vi "Create XY Graph (subVI).vi"(8 "error in":errorcluster caption="error in (no error)", 10 "Direction":dbl[](array[numeric]), 11 "Magnitude":dbl[](array[numeric])) -> (0 "error out":errorcluster, 1 "Polar Array":cluster{dbl, dbl}[](array[cluster]), 3 "XY Graph":cluster{"Y":dbl[], "Y":dbl[]}[](graph))   [LabVIEW 2016]
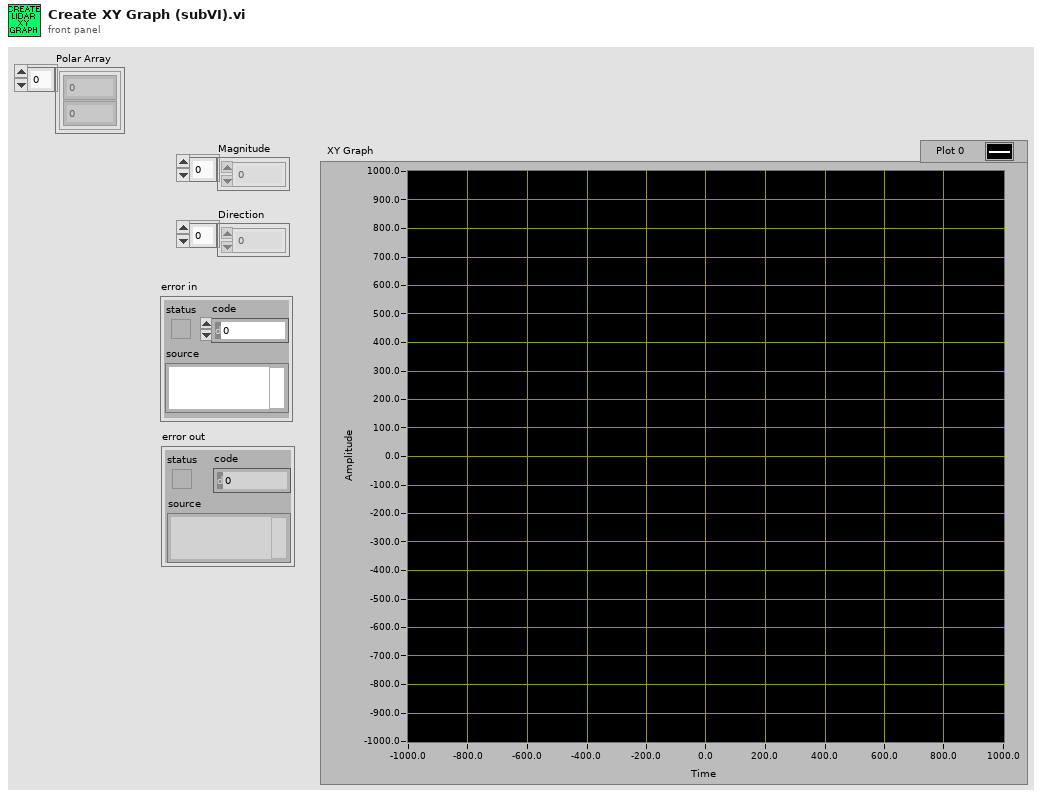
[diagram p1: front panel]
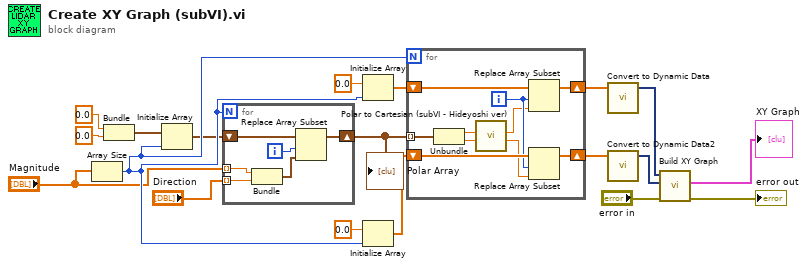
[diagram p0: block diagram]
diagram:
  n1 = Array Size(array="Magnitude") -> (size(s)=w12:i32)
  n2 = Bundle(0.0, 0.0) -> (w5:cluster{dbl, dbl})  [unwired: 1 in]
  n3 = Initialize Array(w5, w12) -> (w6:cluster{dbl, dbl}[])
  n4 = for {
    N: w12 -> [_]
    shift-right: [w21] -> w9
    shift-left: w6 -> [w22]
    tunnel: "Magnitude" -> [w25] mode=indexing
    tunnel: "Direction" -> [w24] mode=indexing
    i -> [w23]
    n5 = Bundle(w25, w24) -> (w20:cluster{dbl, dbl})  [unwired: 1 in]
    n6 = Replace Array Subset(array=w22, new element=w20, index=w23) -> (w21:cluster{dbl, dbl}[])
  }
  "Polar Array" <- w9
  n7 = Initialize Array(0.0 ("element"), w12) -> (w13:dbl[])
  n8 = Initialize Array(0.0 ("element"), w12) -> (w14:dbl[])
  n9 = for {
    N: w12 -> [_]
    tunnel: w9 -> [w35] mode=indexing
    shift-right: [w31] -> w16
    shift-left: w13 -> [w34]
    shift-right: [w30] -> w18
    shift-left: w14 -> [w33]
    i -> [w32]
    n10 = Unbundle(w35) -> (w27:dbl, w26:dbl)
    n11 = call "Polar to Cartesian (subVI - Hideyoshi ver).vi"("Angle (rads)"=w26, "Magnitude (r)"=w27) -> ("y (r*sin(theta))"=w28:dbl, "x (r*cos(theta))"=w29:dbl)  [unwired: 8 in]
    n12 = Replace Array Subset(array=w34, new element=w29, index=w32) -> (w31:dbl[])
    n13 = Replace Array Subset(array=w33, new element=w28, index=w32) -> (w30:dbl[])
  }
  n14 = call "Convert to Dynamic Data"("Array"=w16) -> ("Dynamic Data Type"=w17:dynamicdata)  [unwired: 3 in]
  n15 = call "Convert to Dynamic Data2"("Array"=w18) -> ("Dynamic Data Type"=w19:dynamicdata)  [unwired: 3 in]
  n16 = call "Build XY Graph"("error in (no error)"="error in", "Y Input"=w19, "X Input"=w17) -> ("error out"=→"error out":errorcluster, "XY Graph"=→"XY Graph":cluster{"X":dbl[], "Y":dbl[]}[])  [unwired: 7 in]
